vi "Zedver_v2_write_and_read_once.vi"(0 "connection ID in":refnum<k5>, 2 "data to send":string, 3 "error in":errorcluster) -> (7 "connection ID out":refnum<k5>, 9 "data read":string, 10 "error out":errorcluster)   [LabVIEW 2011]
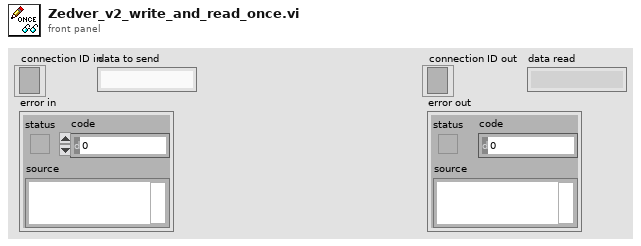
[diagram p1: front panel]
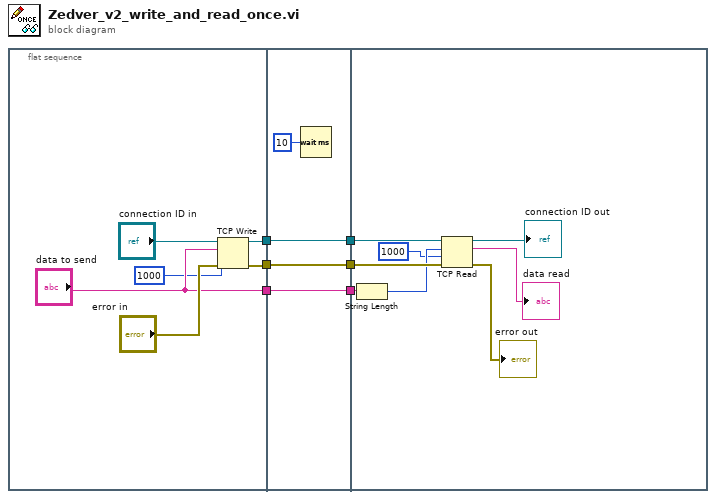
[diagram p0: block diagram]
diagram:
  n1 = flat-sequence {
    tunnel: [w10] -> w6
    tunnel: [w9] -> w4
    tunnel: ["data to send"] -> w2
    tunnel: w6 -> [w16]
    tunnel: [w16] -> w5
    tunnel: w4 -> [w15]
    tunnel: [w15] -> w3
    tunnel: w2 -> [w14]
    tunnel: [w14] -> w1
    tunnel: w5 -> [w22]
    tunnel: w3 -> [w21]
    tunnel: w1 -> [w19]
    frame #0 {
      n2 = TCP Write(connection ID="connection ID in", data in="data to send", error in (no error)="error in", 9:1000 ("timeout ms (25000)")) -> (connection ID out=w10:refnum<k5>, error out=w9:errorcluster)  [unwired: 1 out]
    }
    frame #1 {
      n3 = Wait (ms)(milliseconds to wait=u32 10) -> ()  [unwired: 1 out]
    }
    frame #2 {
      n4 = String Length(string=w19) -> (length=w18:i32)
      n5 = TCP Read(connection ID=w22, bytes to read=w18, error in (no error)=w21, 9:1000 ("timeout ms (25000)")) -> (connection ID out=→"connection ID out":refnum<k5>, data out=→"data read":string, error out=→"error out":errorcluster)  [unwired: 1 in]
    }
  }
